vi "FM Receiver.vi"() -> ()   [LabVIEW 2013]
doc: "Use this template to build a producer/consumer design pattern. Use this template when you need to execute a process, such as data analysis, when a data source, such as a triggered acquisition, produces data at an uneven rate and you need to execute the process when the data becomes available."
uses:
  <vilib>/Waveform/WDTFileIO.llb/Read Waveform from File.vi
  <vilib>/Analysis/NI_AALPro.lvlib
  <vilib>/Analysis/2dsp.llb/Rational Resample (single channel, DBL).vi
  <vilib>/sound2/lvsound2.llb/Sound Output Write (DBL Single).vi
panel:
  out "date string":string
  out "time string":string
  in  "stop":bool
  in  "Name 2":cluster{"Decimation":u32, "Interpolation":u32}
  in  "Sound format":T1
  in  "IQ Rate":u32(slide) scale=0.0..10.0 scale format="%#_6p"
  in  "file path (dialog if empty)":path
  out "Waveform":waveform(dbl)(graph)
  out "error out":errorcluster
  out "error out":errorcluster
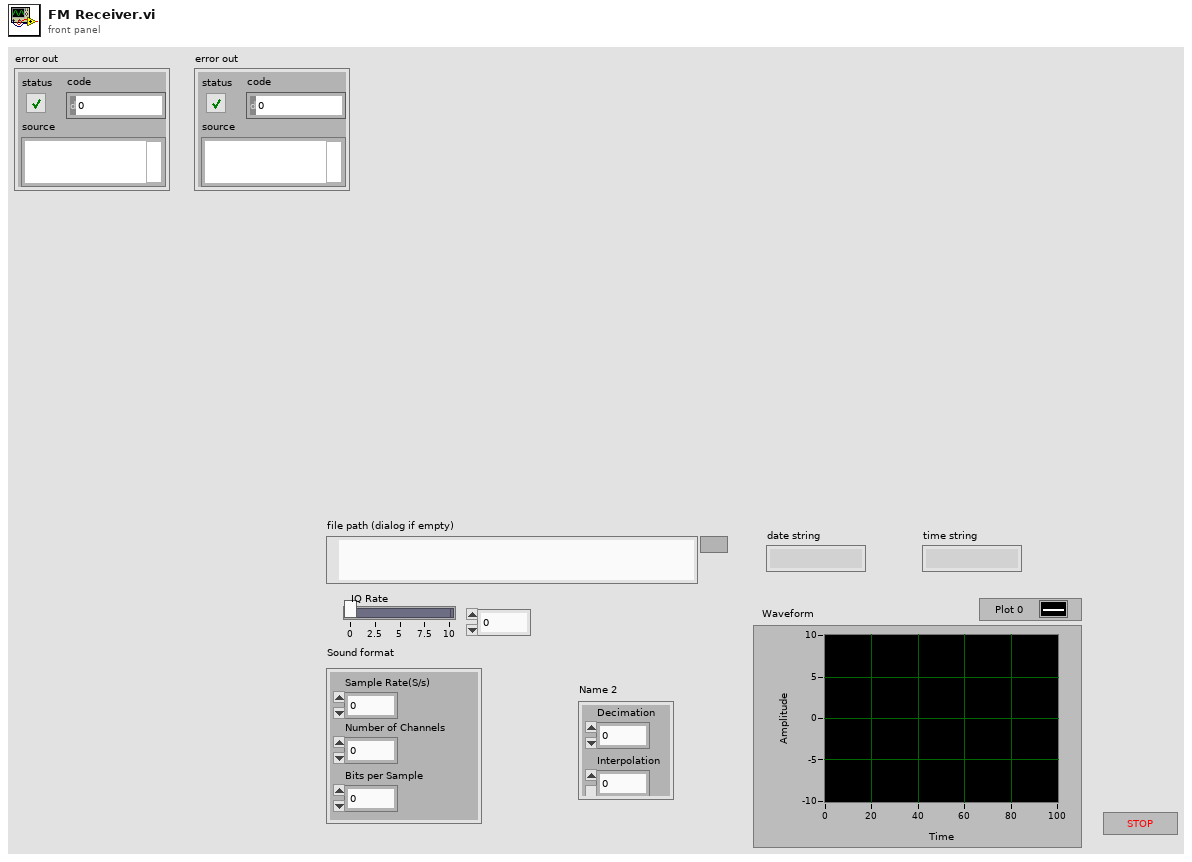
[diagram p1: front panel]
types:
  T1 = cluster{"Sample Rate(S/s)":dbl, "Number of Channels":dbl, "Bits per Sample":dbl}
  T2 = typedef "Sound Output Task ID.ctl" = u32
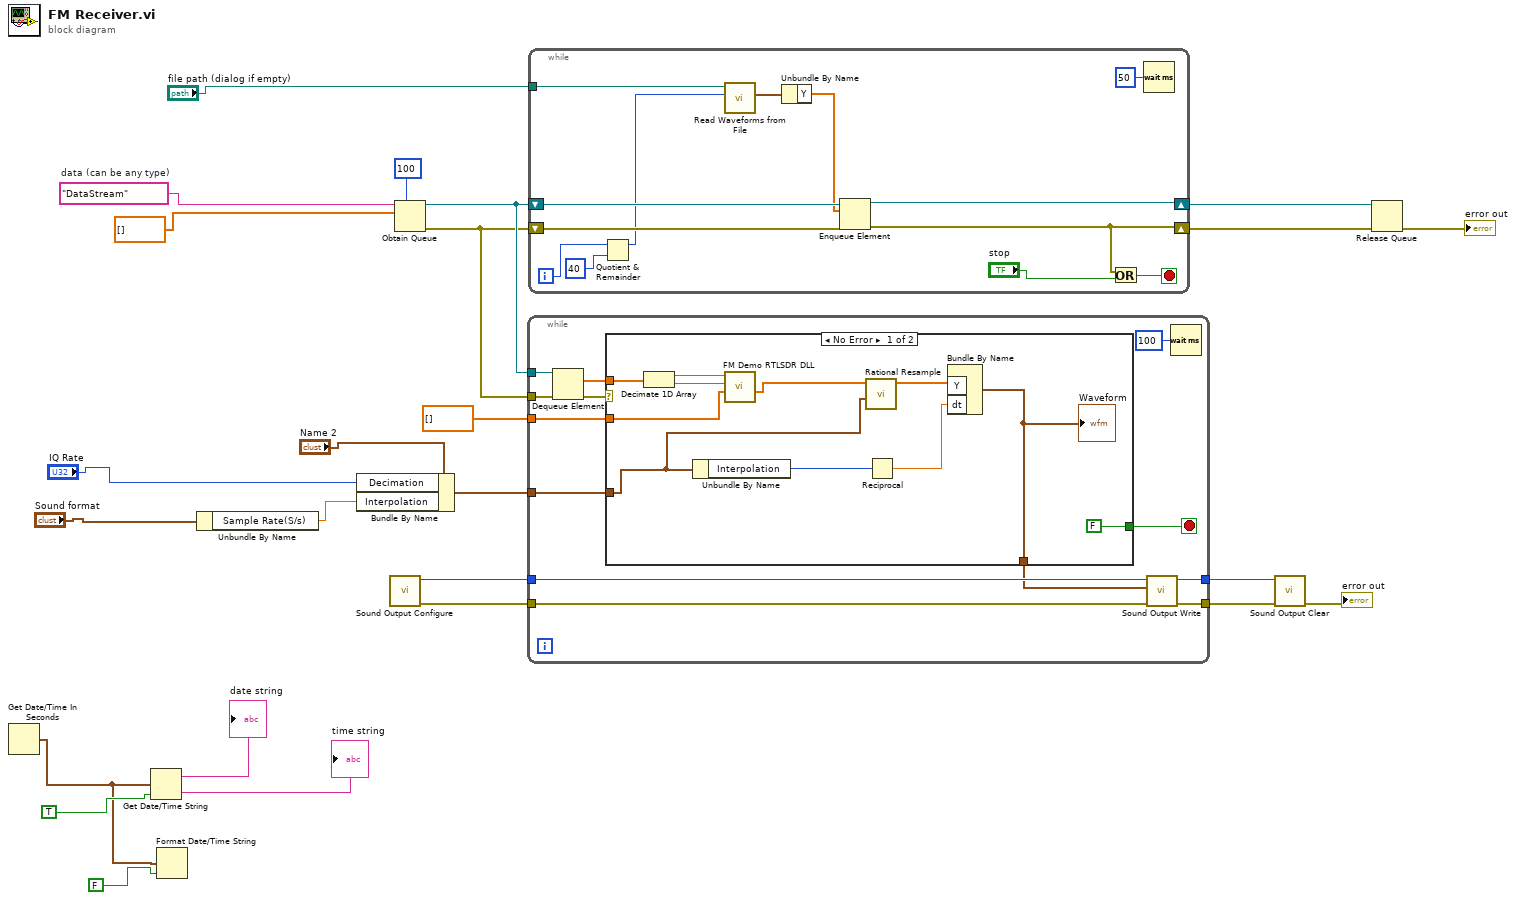
[diagram p0: block diagram]
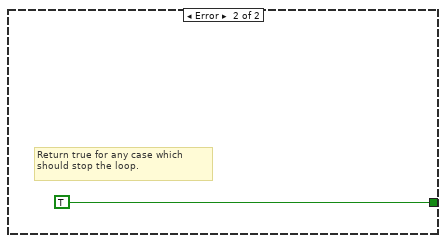
[diagram p2: hidden frame]
diagram:
  w19 = "DataStream"  # data (can be any type)
  n1 = Get Date/Time In Seconds() -> (seconds since 1Jan1904=w3:timestamp)
  n2 = Get Date/Time String(seconds (now)=w3, want seconds? (F)=TRUE) -> (date string=→"date string":string, time string=→"time string":string)  [unwired: 1 in]
  n3 = Format Date/Time String(seconds (now)=w3, UTC format=FALSE) -> ()  [unwired: 1 in, 1 out]
  n4 = Unbundle By Name("Sound format") -> ("Sample Rate(S/s)"=w12:dbl)
  n5 = Bundle By Name(cluster="Name 2", "Decimation"="IQ Rate", "Interpolation"=w12) -> (w10:cluster{"Decimation":u32, "Interpolation":u32})
  n6 = call <vilib>:"Sound Output Configure.vi"() -> ("error out"=w15:errorcluster, "task ID"=w13:T2)  [unwired: 10 in]
  n7 = Obtain Queue(max queue size (-1, unlimited)=100, name (unnamed)=w19, element data type=dbl[] []) -> (queue out=w25:refnum<queue>, error out=w20:errorcluster)  [unwired: 2 in, 1 out]
  n8 = while {
    tunnel: w25 -> [w38]
    tunnel: w20 -> [w34]
    tunnel: [w32] -> w17
    tunnel: [w31] -> w16
    tunnel: w15 -> [w30]
    tunnel: w13 -> [w29]
    tunnel: dbl[] [] -> [w27]
    tunnel: w10 -> [w26]
    stop <- w35 stop-if-true
    n9 = Dequeue Element(queue=w38, error in (no error)=w34) -> (element=w36:dbl[], error out=w37:errorcluster)  [unwired: 1 in, 2 out]
    n10 = case shown="No Error" w37 {
      tunnel: w36 -> [w48 _]
      tunnel: [FALSE TRUE] -> w35
      tunnel: [w39 _] -> w28
      tunnel: w27 -> [w43 _]
      tunnel: w26 -> [w41 _]
      frame No Error {
        n11 = Decimate 1D Array(w48) -> (w45:dbl[], w44:dbl[])
        n12 = Unbundle By Name(w41) -> ("Interpolation"=w40:u32)
        n13 = call <userlib>:"FM Demo RTLSDR DLL.vi"("Baseband"=w43, "QSamples"=w44, "ISamples"=w45) -> ("Baseband out"=w42:dbl[])  [unwired: 8 in]
        n14 = call-poly <vilib>:"Rational Resample.vi"("resample factor"=w41, "X"=w42) -> ("Y"=w47:dbl[])  [unwired: 7 in, 2 out]
        n15 = Reciprocal(x=w40) -> (1/x=w46:dbl)
        n16 = Bundle By Name("Y"=w47, "dt"=w46) -> (w39:waveform(dbl))  [unwired: 1 in]
        "Waveform" <- w39
      }
      frame Error {
        # "Return true for any case which should stop the loop."
      }
    }
    n17 = call-poly <vilib>:"Sound Output Write.vi"("error in (no error)"=w30, "data"=w28, "task ID"=w29) -> ("error out"=w31:errorcluster, "task ID out"=w32:T2)  [unwired: 7 in]
    n18 = Wait (ms)(milliseconds to wait=u32 100) -> ()  [unwired: 1 out]
  }
  n19 = while {
    shift-right: [w52] -> w23
    shift-left: w20 -> [w59]
    shift-right: [w60] -> w24
    shift-left: w25 -> [w58]
    tunnel: "file path (dialog if empty)" -> [w62]
    i -> [w57]
    stop <- w53 stop-if-true
    n20 = Quotient & Remainder(x=w57, y=40) -> (x-y*floor(x/y)=w55:i32)  [unwired: 1 out]
    n21 = call-poly <vilib>:"Read Waveforms from File.vi"("offset (records:0)"=w55, "file path (dialog if empty)"=w62) -> ("first waveform in record"=w61:waveform(dbl))  [unwired: 4 in, 3 out]
    n22 = Unbundle By Name(w61) -> ("Y"=w54:dbl[])
    n23 = Enqueue Element(queue=w58, element=w54, error in (no error)=w59) -> (queue out=w60:refnum<queue>, error out=w52:errorcluster)  [unwired: 1 in, 1 out]
    n24 = Or(x=w52, y="stop") -> (x .or. y?=w53:bool)
    n25 = Wait (ms)(milliseconds to wait=u32 50) -> ()  [unwired: 1 out]
  }
  n26 = call <vilib>:"Sound Output Clear.vi"("error in (no error)"=w16, "task ID"=w17) -> ("error out"=→"error out":errorcluster)  [unwired: 9 in]
  n27 = Release Queue(queue=w24, error in (no error)=w23) -> (error out=→"error out":errorcluster)  [unwired: 1 in, 2 out]
